vi "Teleop.vi"(10 "Match Info":T1={"Autonomous Elapsed Seconds"=0.0, "TeleOp Elapsed Seconds"=0.0, "Disabled Elapsed Seconds"=0.0, "Visited Autonomous"=FALSE, "Visited TeleOp"=FALSE, "Visited Disabled"=FALSE, "Autonomous Settings"={"Autonomous Style"=enum."Independent", "VI Refnum"=refnum}}, 11 "Call Context":T2) -> ()   [LabVIEW 2017]
doc: "This VI is called for each TeleOp packet received from the DS where the robot is not disabled. It is often used to read from the joysticks and update I/O or to update setpoints for timed control loops. It should complete and return within 20 milliseconds or it may miss DS packets."
uses:
  <vilib>/Rock Robotics/WPI/DriverStation/WPI_DriverStationDerivedRobotMode.ctl
  <vilib>/Rock Robotics/WPI/DriverStation/WPI_DriverStationMatch Info.ctl
  _SHARE ALL/TypeDef Share All/ENUM_Joystick_Buttons.ctl
  _SHARE ALL/TypeDef Share All/ENUM_Joystick_Axes.ctl
  _SHARE ALL/RoboRio Share All/Systems Share All/Joystick/Global_Joystick Write_Data.vi
  Globals/CMD_Global.vi
  _SHARE ALL/RoboRio Share All/Systems Share All/Joystick/Joystick.lvlib
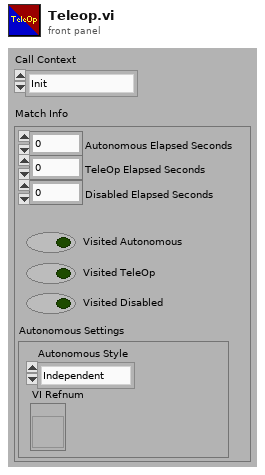
[diagram p1: front panel]
types:
  T1 = typedef "WPI_DriverStationMatch Info.ctl" = cluster{"Autonomous Elapsed Seconds":dbl, "TeleOp Elapsed Seconds":dbl, "Disabled Elapsed Seconds":dbl, "Visited Autonomous":bool, "Visited TeleOp":bool, "Visited Disabled":bool, "Autonomous Settings":cluster{"Autonomous Style":enum16{"Iterative", "Independent"}, "VI Refnum":refnum<vi>}}
  T2 = typedef "WPI_DriverStationDerivedRobotMode.ctl" = enum16{"Init", "Execute", "Stop"}
  T3 = typedef "ENUM_Joystick_Axes.ctl" = enum16{"Left X", "Left Y", "Left Trigger", "Right Trigger", "Right X", "Right Y"}
  T4 = typedef "ENUM_Joystick_Buttons.ctl" = enum16{"Green A", "Red B", "Blue X", "Yellow Y", "Left Bumper", "Right Bumper", "Back", "Start", "Left Joystick", "Right Joystick"}
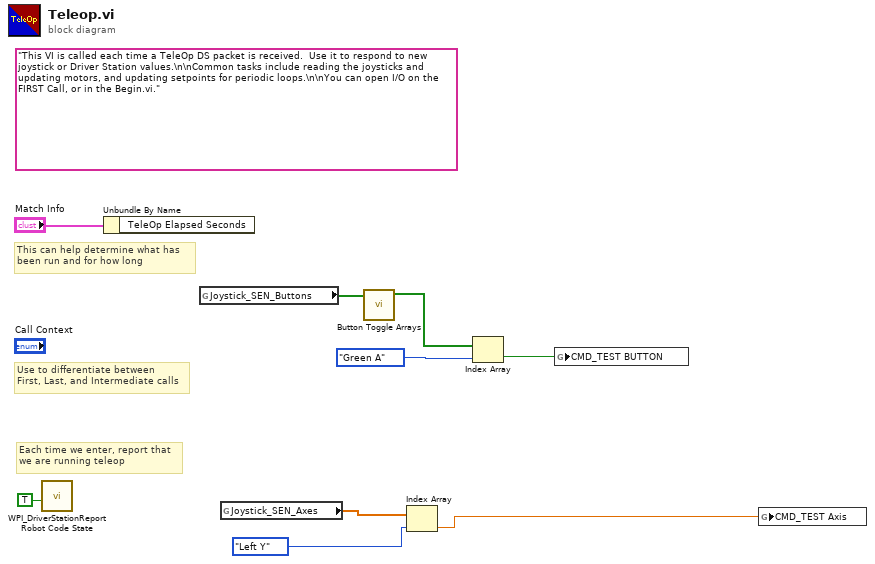
[diagram p0: block diagram]
diagram:
  (unwired) "This VI is called each time a TeleOp DS packet is received.  Use it to respond to new joystick or Driver Station values.\n\nCommon tasks include reading the joysticks and updating motors, and updating setpoints for periodic loops.\n\nYou can open I/O on the FIRST Call, or in the Begin.vi."
  # "Each time we enter, report that\nwe are running teleop"
  # "Use to differentiate between\nFirst, Last, and Intermediate calls"
  # "This can help determine what has\nbeen run and for how long"
  n1 = call <vilib>:"WPI_DriverStationReport Robot Code State.vi"("TeleOp"=TRUE ("Autonomous")) -> ()  [unwired: 10 in, 1 out]
  n2 = Unbundle By Name("Match Info") -> ()  [unwired: 1 out]
  n3 = global read "Global_Joystick Write_Data.vi" "Joystick_SEN_Buttons"() -> (w4:bool[])
  n4 = global read "Global_Joystick Write_Data.vi" "Joystick_SEN_Axes"() -> (w6:dbl[])
  n5 = call "Button Toggle Arrays.vi"("Joystick_SEN_Buttons"=w4) -> ("Toggle Outputs Out"=w3:bool[])  [unwired: 8 in, 2 out]
  n6 = Index Array(array=w6, index=ENUM_Joystick_Axes."Left Y") -> (element=w2:dbl)
  n7 = Index Array(array=w3, index=ENUM_Joystick_Buttons."Green A") -> (element=w1:bool)
  n8 = global write "CMD_Global.vi" "CMD_TEST BUTTON"(w1) -> ()
  n9 = global write "CMD_Global.vi" "CMD_TEST Axis"(w2) -> ()
